vi "配置文件保存.vi"   [LabVIEW 2016, in "斯坦道总氮.lvlib"]
uses:
  <vilib>/Utility/config.llb/NI_LVConfig.lvlib
types:
  T1 = typedef "NI_LVConfig.lvlib/Config Data RefNum.ctl" = refnum<k1>
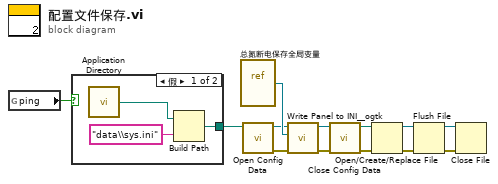
[diagram p0: block diagram]
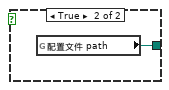
[diagram p2: hidden frame]
diagram:
  n1 = global read "VAR总氮全局变量.vi" "ping"() -> (w2:bool)
  n2 = case shown="假" w2 {
    tunnel: [w15 w17] -> w1
    frame False {
      n3 = call <vilib>:"Application Directory.vi"() -> ("Application Directory"=w14:path)
      n4 = Build Path(base path=w14, name or relative path="data\\sys.ini" ("名称或相对路径")) -> (appended path=w15:path)
    }
    frame True {
      n5 = global read "VAR总氮全局变量.vi" "配置文件 path"() -> (w17:path)
    }
  }
  n6 = vi-ref "总氮断电保存全局变量.vi"() -> (w4:refnum<vi>)
  n7 = call <vilib>:"Open Config Data.vi"("configuration file path"=w1) -> ("error out"=w6:errorcluster, "refnum"=w3:T1)  [unwired: 8 in, 1 out]
  n8 = call <userlib>:"Write Panel to INI__ogtk.vi"("error in (no error)"=w6, "VI ref"=w4, "refnum"=w3) -> ("error out"=w7:errorcluster, "refnum out"=w5:T1)  [unwired: 7 in]
  n9 = call <vilib>:"Close Config Data.vi"("error in (no error)"=w7, "refnum"=w5) -> ("error out"=w12:errorcluster, "file path"=w13:path)  [unwired: 8 in]
  n10 = Open/Create/Replace File(file path (use dialog)=w13, error in=w12) -> (refnum out=w9:refnum<file>, error out=w8:errorcluster)  [unwired: 4 in, 1 out]
  n11 = Flush File(refnum=w9, error in=w8) -> (refnum out=w10:refnum<file>, error out=w11:errorcluster)
  n12 = Close File(refnum=w10, error in=w11) -> ()  [unwired: 2 out]
